vi "writeToXML.vi"(8 "error in (no error)":errorcluster, 10 "ClassLabel":string, 11 "TCSTcsCommand in":refnum<class "TCSTcsCommand.lvclass">) -> (0 "error out":errorcluster, 2 "XML out":string, 3 "TCSTcsCommand out":refnum<class "TCSTcsCommand.lvclass">)   [LabVIEW 2022 SP3, in "TCSDataDefinitions.lvlib" / "TCSCommand.lvlib" / "TCSTcsCommand.lvclass"]
uses:
  TCSTcsCommand.lvclass
  TCSCommand/TCSCommand.lvclass
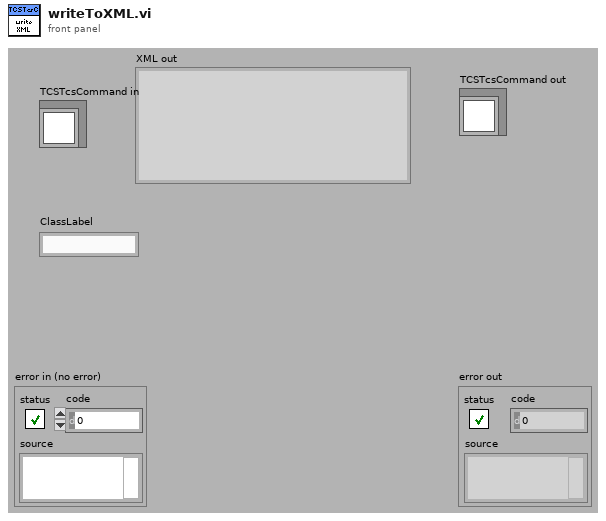
[diagram p1: front panel]
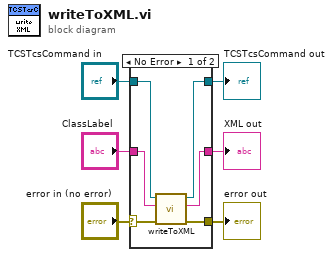
[diagram p0: block diagram]
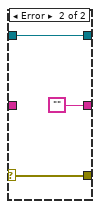
[diagram p2: hidden frame]
diagram:
  n1 = case shown="No Error" "error in (no error)" {
    selector: "error in (no error)" -> [w8 w15]
    tunnel: [w7 w15] -> w5
    tunnel: [w10 w14] -> w2
    tunnel: "TCSTcsCommand in" -> [w11 w14]
    tunnel: "ClassLabel" -> [w12 _]
    tunnel: [w9 ""] -> w3
    frame No Error {
      n2 = call-parent "writeToXML.vi"("error in (no error)"=w8, "Class Label"=w12, "TCSCommand in"=w11) -> ("error out"=w7:errorcluster, "XML out"=w9:string, "TCSCommand out"=w10:refnum<class "TCSTcsCommand.lvclass">)  [unwired: 6 in]
    }
    frame Error {
    }
  }
  "error out" <- w5
  "XML out" <- w3
  "TCSTcsCommand out" <- w2
